vi "FFT Software Example.vi"() -> ()   [LabVIEW 2014]
doc: "Tested with:\n - Wemos D1 with ESP8266\nNot running on Arduino Nano due to not enough RAM, program compile and upload but don't output results (probably crash during computation, arduino has no floating point unit)\n\nSoftware implementation of FFT. It's running in simulation mode on desktop PC and also on MCU."
uses:
  <vilib>/LabVIEW Universal Transcriptor/LabVIEW to Arduino Transcriptor/Transcriptors/System API/Serial println string.vi
  <vilib>/LabVIEW Universal Transcriptor/LabVIEW for Arduino Complex Numbers Static/ComplexNumberStatic.lvclass
  LabVIEW-Universal-Transcriptor/Transcriptors/System API/System Serial Library Variables/System Serial Library Variables.lvlib
panel:
  out "FFT signal spectrum":dbl[](graph)
  out "String Buffer":string
  out "error out":errorcluster
  in  "error in":errorcluster
  out "Input Signal":dbl[](graph)
  # "Implementation of diagram of FFT. I redraw it into LabVIEW just to see\nif it's really true how they say :D And YES, it's true.\n\nTHIS EXAMPLE IS JUST FOR ESP8266, IT'S NOT RUNNING ON Arduino NOT BECAUSE WRON PROGRAM, BUT IT HAS NOT ENOUGHT COMPUTATION POWER, PROBABLY IT'S SILENTLY CRASHING DURING COMPUTATION OR SOMETHING ELSE."
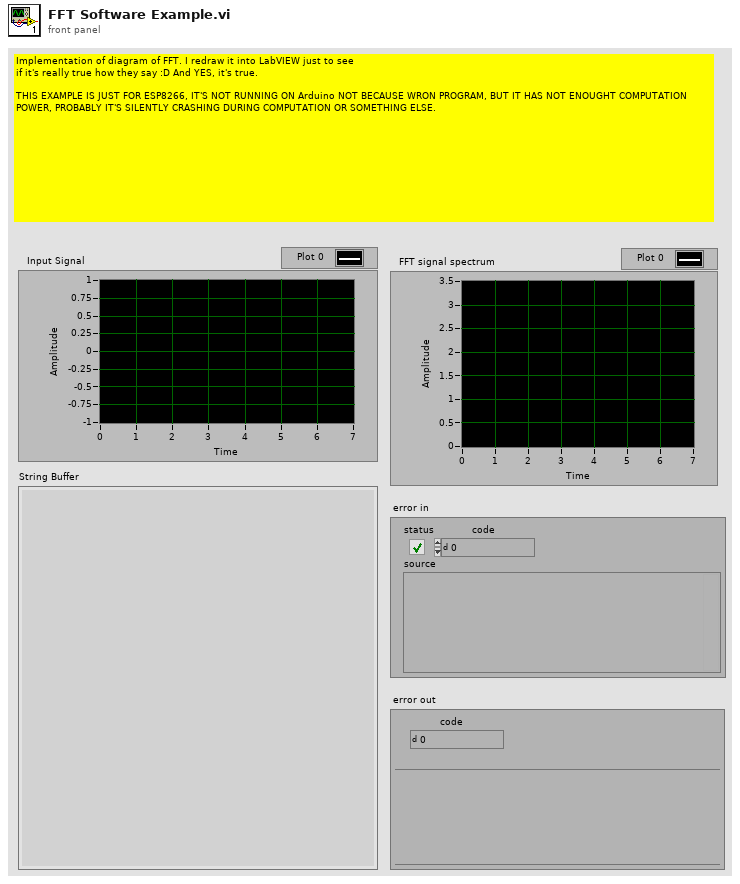
[diagram p1: front panel]
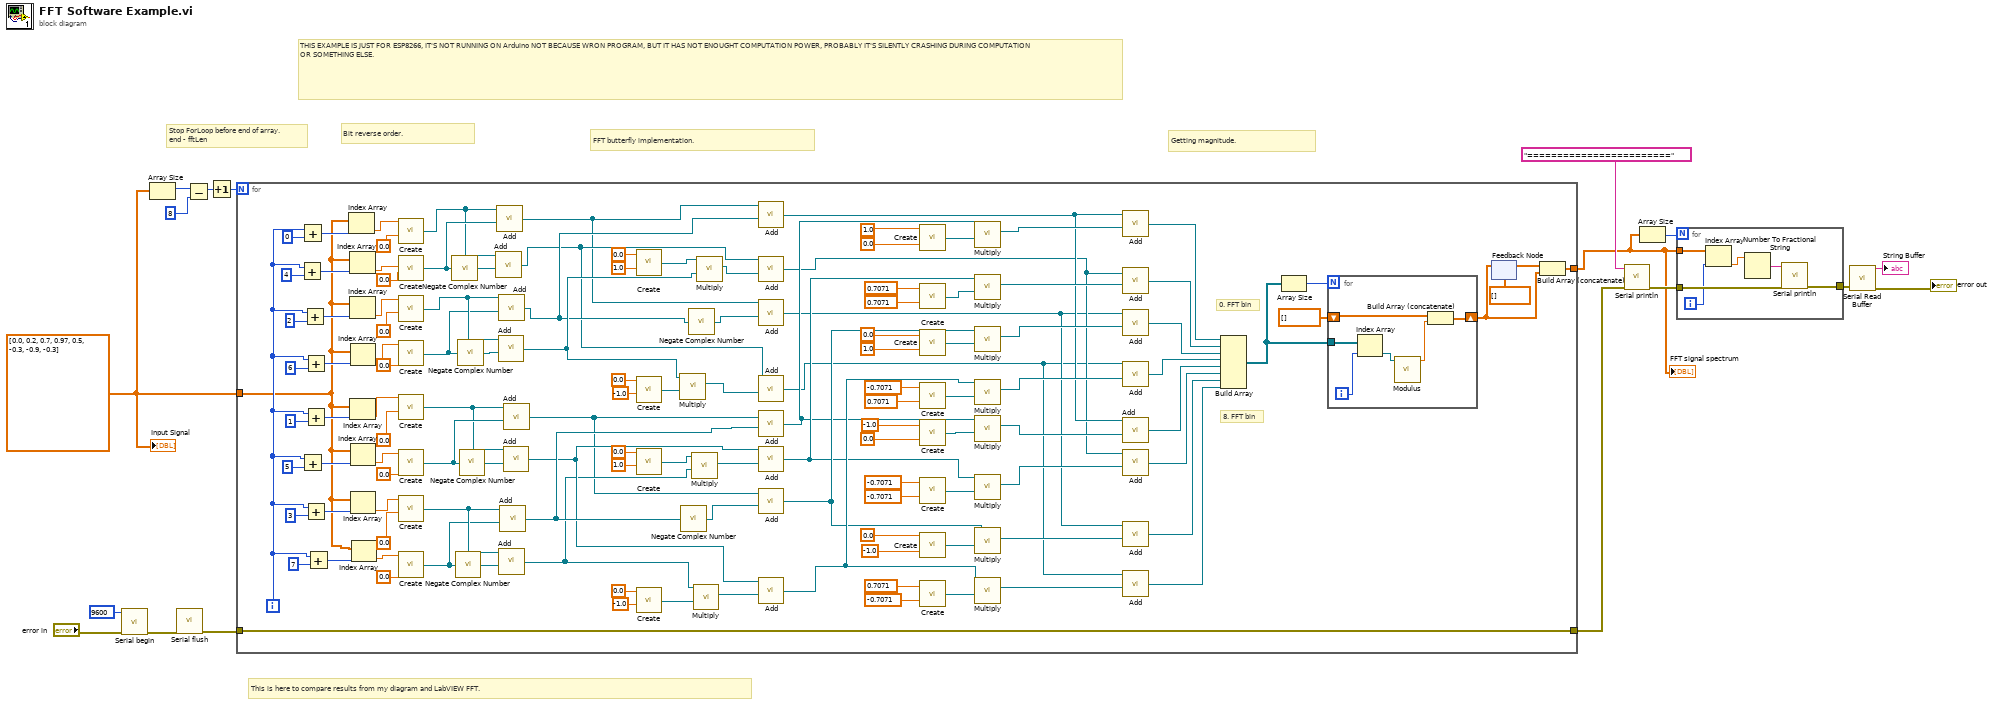
[diagram p0: block diagram]
diagram:
  w14 = dbl[] [0.0, 0.2, 0.7, 0.97, 0.5, -0.3, -0.9, -0.3] ("Y")
  # "THIS EXAMPLE IS JUST FOR ESP8266, IT'S NOT RUNNING ON Arduino NOT BECAUSE WRON PROGRAM, BUT IT HAS NOT ENOUGHT COMPUTATION POWER, PROBABLY IT'S SILENTLY CRASHING DURING COMPUTATION OR SOMETHING ELSE."
  # "Stop ForLoop before end of array.\nend - fftLen"
  # "Getting magnitude."
  # "Bit reverse order."
  # "This is here to compare results from my diagram and LabVIEW FFT."
  # "FFT butterfly implementation."
  n1 = call <vilib>:"Serial begin.vi"("Error In"="error in", "speed (Bd)"=9600) -> ("Error Out"=w4:errorcluster)  [unwired: 9 in]
  n2 = Array Size(array=w14) -> (size(s)=w16:i32)
  n3 = call <vilib>:"Serial flush.vi"("Error In"=w4) -> ("Error Out"=w3:errorcluster)  [unwired: 10 in]
  n4 = Subtract(x=w16, y=8) -> (x-y=w17:i32)
  n5 = Increment(x=w17) -> (x+1=w1:i32)
  n6 = for {
    N: w1 -> [_]
    tunnel: w14 -> [w18]
    tunnel: [w23] -> w2
    tunnel: w3 -> [w20]
    tunnel: [w20] -> w12
    i -> [w129]
    # "8. FFT bin"
    # "0. FFT bin"
    n7 = Add(x=w129, y=4) -> (x+y=w142:i32)
    n8 = Add(x=w129, y=0) -> (x+y=w145:i32)
    n9 = Add(x=w129, y=5) -> (x+y=w136:i32)
    n10 = Add(x=w129, y=2) -> (x+y=w140:i32)
    n11 = Add(x=w129, y=6) -> (x+y=w130:i32)
    n12 = Add(x=w129, y=1) -> (x+y=w131:i32)
    n13 = Add(x=w129, y=3) -> (x+y=w134:i32)
    n14 = Add(x=w129, y=7) -> (x+y=w132:i32)
    n15 = Index Array(array=w18, index=w145) -> (element=w127:dbl)
    n16 = Index Array(array=w18, index=w142) -> (element=w125:dbl)
    n17 = Index Array(array=w18, index=w140) -> (element=w115:dbl)
    n18 = Index Array(array=w18, index=w131) -> (element=w109:dbl)
    n19 = Index Array(array=w18, index=w130) -> (element=w116:dbl)
    n20 = Index Array(array=w18, index=w136) -> (element=w108:dbl)
    n21 = Index Array(array=w18, index=w134) -> (element=w102:dbl)
    n22 = Index Array(array=w18, index=w132) -> (element=w101:dbl)
    n23 = call <vilib>:"Create.vi"("Imag"=0.0 ("y"), "Real"=w127) -> ("ComplexNumber"=w122:refnum<class "ComplexNumberStatic.lvclass">)  [unwired: 3 in, 1 out]
    n24 = call <vilib>:"Create.vi"("Imag"=0.0 ("y"), "Real"=w125) -> ("ComplexNumber"=w124:refnum<class "ComplexNumberStatic.lvclass">)  [unwired: 3 in, 1 out]
    n25 = call <vilib>:"Create.vi"("Imag"=0.0 ("y"), "Real"=w115) -> ("ComplexNumber"=w121:refnum<class "ComplexNumberStatic.lvclass">)  [unwired: 3 in, 1 out]
    n26 = call <vilib>:"Create.vi"("Imag"=0.0 ("y"), "Real"=w116) -> ("ComplexNumber"=w119:refnum<class "ComplexNumberStatic.lvclass">)  [unwired: 3 in, 1 out]
    n27 = call <vilib>:"Create.vi"("Imag"=0.0 ("y"), "Real"=w109) -> ("ComplexNumber"=w110:refnum<class "ComplexNumberStatic.lvclass">)  [unwired: 3 in, 1 out]
    n28 = call <vilib>:"Create.vi"("Imag"=0.0 ("y"), "Real"=w108) -> ("ComplexNumber"=w112:refnum<class "ComplexNumberStatic.lvclass">)  [unwired: 3 in, 1 out]
    n29 = call <vilib>:"Create.vi"("Imag"=0.0 ("y"), "Real"=w102) -> ("ComplexNumber"=w107:refnum<class "ComplexNumberStatic.lvclass">)  [unwired: 3 in, 1 out]
    n30 = call <vilib>:"Create.vi"("Imag"=0.0 ("y"), "Real"=w101) -> ("ComplexNumber"=w105:refnum<class "ComplexNumberStatic.lvclass">)  [unwired: 3 in, 1 out]
    n31 = call "Negate Complex Number.vi"("ComplexNumber in"=w124) -> ("ComplexNumber out"=w123:refnum<class "ComplexNumberStatic.lvclass">)
    n32 = call "Negate Complex Number.vi"("ComplexNumber in"=w105) -> ("ComplexNumber out"=w106:refnum<class "ComplexNumberStatic.lvclass">)
    n33 = call "Negate Complex Number.vi"("ComplexNumber in"=w119) -> ("ComplexNumber out"=w120:refnum<class "ComplexNumberStatic.lvclass">)
    n34 = call "Negate Complex Number.vi"("ComplexNumber in"=w112) -> ("ComplexNumber out"=w111:refnum<class "ComplexNumberStatic.lvclass">)
    n35 = call <vilib>:"Add.vi"("A"=w122, "B"=w123) -> ("A+B"=w88:refnum<class "ComplexNumberStatic.lvclass">)  [unwired: 5 in, 1 out]
    n36 = call <vilib>:"Add.vi"("A"=w122, "B"=w124) -> ("A+B"=w76:refnum<class "ComplexNumberStatic.lvclass">)  [unwired: 5 in, 1 out]
    n37 = call <vilib>:"Add.vi"("A"=w121, "B"=w120) -> ("A+B"=w90:refnum<class "ComplexNumberStatic.lvclass">)  [unwired: 5 in, 1 out]
    n38 = call <vilib>:"Add.vi"("A"=w121, "B"=w119) -> ("A+B"=w89:refnum<class "ComplexNumberStatic.lvclass">)  [unwired: 5 in, 1 out]
    n39 = call <vilib>:"Add.vi"("A"=w107, "B"=w106) -> ("A+B"=w78:refnum<class "ComplexNumberStatic.lvclass">)  [unwired: 5 in, 1 out]
    n40 = call <vilib>:"Add.vi"("A"=w107, "B"=w105) -> ("A+B"=w83:refnum<class "ComplexNumberStatic.lvclass">)  [unwired: 5 in, 1 out]
    n41 = call <vilib>:"Add.vi"("A"=w110, "B"=w111) -> ("A+B"=w79:refnum<class "ComplexNumberStatic.lvclass">)  [unwired: 5 in, 1 out]
    n42 = call <vilib>:"Add.vi"("A"=w110, "B"=w112) -> ("A+B"=w77:refnum<class "ComplexNumberStatic.lvclass">)  [unwired: 5 in, 1 out]
    n43 = call <vilib>:"Create.vi"("Imag"=1.0, "Real"=0.0) -> ("ComplexNumber"=w94:refnum<class "ComplexNumberStatic.lvclass">)  [unwired: 3 in, 1 out]
    n44 = call <vilib>:"Create.vi"("Imag"=-1.0, "Real"=0.0) -> ("ComplexNumber"=w96:refnum<class "ComplexNumberStatic.lvclass">)  [unwired: 3 in, 1 out]
    n45 = call <vilib>:"Create.vi"("Imag"=1.0, "Real"=0.0) -> ("ComplexNumber"=w85:refnum<class "ComplexNumberStatic.lvclass">)  [unwired: 3 in, 1 out]
    n46 = call <vilib>:"Create.vi"("Imag"=-1.0, "Real"=0.0) -> ("ComplexNumber"=w82:refnum<class "ComplexNumberStatic.lvclass">)  [unwired: 3 in, 1 out]
    n47 = call <vilib>:"Multiply.vi"("B"=w96, "A"=w90) -> ("A*B"=w95:refnum<class "ComplexNumberStatic.lvclass">)  [unwired: 8 in, 1 out]
    n48 = call "Negate Complex Number.vi"("ComplexNumber in"=w83) -> ("ComplexNumber out"=w100:refnum<class "ComplexNumberStatic.lvclass">)
    n49 = call "Negate Complex Number.vi"("ComplexNumber in"=w89) -> ("ComplexNumber out"=w99:refnum<class "ComplexNumberStatic.lvclass">)
    n50 = call <vilib>:"Multiply.vi"("B"=w78, "A"=w85) -> ("A*B"=w84:refnum<class "ComplexNumberStatic.lvclass">)  [unwired: 8 in, 1 out]
    n51 = call <vilib>:"Multiply.vi"("B"=w82, "A"=w78) -> ("A*B"=w80:refnum<class "ComplexNumberStatic.lvclass">)  [unwired: 8 in, 1 out]
    n52 = call <vilib>:"Multiply.vi"("B"=w90, "A"=w94) -> ("A*B"=w91:refnum<class "ComplexNumberStatic.lvclass">)  [unwired: 8 in, 1 out]
    n53 = call <vilib>:"Add.vi"("A"=w76, "B"=w89) -> ("A+B"=w39:refnum<class "ComplexNumberStatic.lvclass">)  [unwired: 5 in, 1 out]
    n54 = call <vilib>:"Add.vi"("A"=w88, "B"=w91) -> ("A+B"=w36:refnum<class "ComplexNumberStatic.lvclass">)  [unwired: 5 in, 1 out]
    n55 = call <vilib>:"Add.vi"("A"=w76, "B"=w99) -> ("A+B"=w32:refnum<class "ComplexNumberStatic.lvclass">)  [unwired: 5 in, 1 out]
    n56 = call <vilib>:"Add.vi"("A"=w88, "B"=w95) -> ("A+B"=w30:refnum<class "ComplexNumberStatic.lvclass">)  [unwired: 5 in, 1 out]
    n57 = call <vilib>:"Add.vi"("A"=w77, "B"=w83) -> ("A+B"=w48:refnum<class "ComplexNumberStatic.lvclass">)  [unwired: 5 in, 1 out]
    n58 = call <vilib>:"Add.vi"("A"=w79, "B"=w84) -> ("A+B"=w52:refnum<class "ComplexNumberStatic.lvclass">)  [unwired: 5 in, 1 out]
    n59 = call <vilib>:"Add.vi"("A"=w77, "B"=w100) -> ("A+B"=w56:refnum<class "ComplexNumberStatic.lvclass">)  [unwired: 5 in, 1 out]
    n60 = call <vilib>:"Add.vi"("A"=w79, "B"=w80) -> ("A+B"=w59:refnum<class "ComplexNumberStatic.lvclass">)  [unwired: 5 in, 1 out]
    n61 = call <vilib>:"Create.vi"("Imag"=0.0, "Real"=1.0) -> ("ComplexNumber"=w51:refnum<class "ComplexNumberStatic.lvclass">)  [unwired: 3 in, 1 out]
    n62 = call <vilib>:"Create.vi"("Imag"=0.7071, "Real"=0.7071) -> ("ComplexNumber"=w53:refnum<class "ComplexNumberStatic.lvclass">)  [unwired: 3 in, 1 out]
    n63 = call <vilib>:"Create.vi"("Imag"=1.0, "Real"=0.0) -> ("ComplexNumber"=w58:refnum<class "ComplexNumberStatic.lvclass">)  [unwired: 3 in, 1 out]
    n64 = call <vilib>:"Create.vi"("Imag"=0.7071, "Real"=-0.7071) -> ("ComplexNumber"=w60:refnum<class "ComplexNumberStatic.lvclass">)  [unwired: 3 in, 1 out]
    n65 = call <vilib>:"Create.vi"("Imag"=0.0, "Real"=-1.0) -> ("ComplexNumber"=w65:refnum<class "ComplexNumberStatic.lvclass">)  [unwired: 3 in, 1 out]
    n66 = call <vilib>:"Create.vi"("Imag"=-0.7071, "Real"=-0.7071) -> ("ComplexNumber"=w66:refnum<class "ComplexNumberStatic.lvclass">)  [unwired: 3 in, 1 out]
    n67 = call <vilib>:"Create.vi"("Imag"=-1.0, "Real"=0.0) -> ("ComplexNumber"=w70:refnum<class "ComplexNumberStatic.lvclass">)  [unwired: 3 in, 1 out]
    n68 = call <vilib>:"Create.vi"("Imag"=-0.7071, "Real"=0.7071) -> ("ComplexNumber"=w74:refnum<class "ComplexNumberStatic.lvclass">)  [unwired: 3 in, 1 out]
    n69 = call <vilib>:"Multiply.vi"("B"=w51, "A"=w48) -> ("A*B"=w47:refnum<class "ComplexNumberStatic.lvclass">)  [unwired: 8 in, 1 out]
    n70 = call <vilib>:"Multiply.vi"("B"=w53, "A"=w52) -> ("A*B"=w45:refnum<class "ComplexNumberStatic.lvclass">)  [unwired: 8 in, 1 out]
    n71 = call <vilib>:"Multiply.vi"("B"=w58, "A"=w56) -> ("A*B"=w42:refnum<class "ComplexNumberStatic.lvclass">)  [unwired: 8 in, 1 out]
    n72 = call <vilib>:"Multiply.vi"("B"=w60, "A"=w59) -> ("A*B"=w41:refnum<class "ComplexNumberStatic.lvclass">)  [unwired: 8 in, 1 out]
    n73 = call <vilib>:"Multiply.vi"("B"=w65, "A"=w48) -> ("A*B"=w38:refnum<class "ComplexNumberStatic.lvclass">)  [unwired: 8 in, 1 out]
    n74 = call <vilib>:"Multiply.vi"("B"=w66, "A"=w52) -> ("A*B"=w35:refnum<class "ComplexNumberStatic.lvclass">)  [unwired: 8 in, 1 out]
    n75 = call <vilib>:"Multiply.vi"("B"=w70, "A"=w56) -> ("A*B"=w33:refnum<class "ComplexNumberStatic.lvclass">)  [unwired: 8 in, 1 out]
    n76 = call <vilib>:"Multiply.vi"("B"=w74, "A"=w59) -> ("A*B"=w29:refnum<class "ComplexNumberStatic.lvclass">)  [unwired: 8 in, 1 out]
    n77 = call <vilib>:"Add.vi"("A"=w39, "B"=w47) -> ("A+B"=w46:refnum<class "ComplexNumberStatic.lvclass">)  [unwired: 5 in, 1 out]
    n78 = call <vilib>:"Add.vi"("A"=w36, "B"=w45) -> ("A+B"=w44:refnum<class "ComplexNumberStatic.lvclass">)  [unwired: 5 in, 1 out]
    n79 = call <vilib>:"Add.vi"("A"=w32, "B"=w42) -> ("A+B"=w43:refnum<class "ComplexNumberStatic.lvclass">)  [unwired: 5 in, 1 out]
    n80 = call <vilib>:"Add.vi"("A"=w30, "B"=w41) -> ("A+B"=w40:refnum<class "ComplexNumberStatic.lvclass">)  [unwired: 5 in, 1 out]
    n81 = call <vilib>:"Add.vi"("A"=w39, "B"=w38) -> ("A+B"=w37:refnum<class "ComplexNumberStatic.lvclass">)  [unwired: 5 in, 1 out]
    n82 = call <vilib>:"Add.vi"("A"=w36, "B"=w35) -> ("A+B"=w34:refnum<class "ComplexNumberStatic.lvclass">)  [unwired: 5 in, 1 out]
    n83 = call <vilib>:"Add.vi"("A"=w32, "B"=w33) -> ("A+B"=w31:refnum<class "ComplexNumberStatic.lvclass">)  [unwired: 5 in, 1 out]
    n84 = call <vilib>:"Add.vi"("A"=w30, "B"=w29) -> ("A+B"=w28:refnum<class "ComplexNumberStatic.lvclass">)  [unwired: 5 in, 1 out]
    n85 = Build Array(w46, w44, w43, w40, w37, w34, w31, w28) -> (w21:refnum<class "ComplexNumberStatic.lvclass">[])
    n86 = Array Size(array=w21) -> (size(s)=w22:i32)
    n87 = for {
      N: w22 -> [_]
      tunnel: w21 -> [w150]
      shift-right: [w148] -> w25
      shift-left: dbl[] [] -> [w149]
      i -> [w151]
      n88 = Index Array(array=w150, index=w151) -> (element=w147:refnum<class "ComplexNumberStatic.lvclass">)
      n89 = call <vilib>:"Modulus.vi"("A"=w147) -> ("modul"=w146:dbl)  [unwired: 9 in, 1 out]
      n90 = Build Array (concatenate)(w149, w146) -> (w148:dbl[])
    }
    n91 = feedback-in #1(w25) -> ()
    n92 = feedback #1(dbl[] []) -> (w26:dbl[])
    n93 = Build Array (concatenate)(w26, w25) -> (w23:dbl[])
  }
  "FFT signal spectrum" <- w2
  n94 = call-poly <vilib>:"Serial println.vi"("Error In"=w12, "string in"="========================") -> ("Error Out"=w11:errorcluster)  [unwired: 9 in]
  n95 = Array Size(array=w2) -> (size(s)=w10:i32)
  n96 = for {
    N: w10 -> [_]
    tunnel: w11 -> [w157]
    tunnel: w2 -> [w156]
    tunnel: [w152] -> w7
    i -> [w155]
    n97 = Index Array(array=w156, index=w155) -> (element=w154:dbl)
    n98 = Number To Fractional String(number=w154) -> (F-format string=w153:string)  [unwired: 3 in]
    n99 = call-poly <vilib>:"Serial println.vi"("Error In"=w157, "string in"=w153) -> ("Error Out"=w152:errorcluster)  [unwired: 9 in]
  }
  n100 = call <vilib>:"Serial Read Buffer.vi"("Error In"=w7) -> ("Error Out"=→"error out":errorcluster, "String Buffer"=→"String Buffer":string)  [unwired: 9 in]
  "Input Signal" <- w14
